vi "_read_mixer_params.vi"(10 "Control":T1={"GPIB_ATT"="28", "6501Dev#"=1, "GPIB_SP"="18", "GPIB_PM"="13", "GPIB_DSA"="11", "GPIB_DMM (TPD)"="23", "GPIB_MPI"="2", "mortor設定"=[{"Axis"=0, "ID"=0, "HIspeed"=200.0, "LOspeed"=100.0, "ACCEL(ms)"=100.0, "Sratio"=50.0, "フリーラン\n"=FALSE, "文字列"="DSB HOT/COLD"}, {"Axis"=1, "ID"=0, "HIspeed"=4.0, "LOspeed"=4.0, "ACCEL(ms)"=100.0, "Sratio"=50.0, "フリーラン\n"=TRUE, "文字列"="SubMM Att"}, {"Axis"=0, "ID"=0, "HIspeed"=200.0, "LOspeed"=100.0, "ACCEL(ms)"=100.0, "Sratio"=50.0, "フリーラン\n"=TRUE, "文字列"="MPI Port1"}, {"Axis"=1, "ID"=0, "HIspeed"=200.0, "LOspeed"=100.0, "ACCEL(ms)"=100.0, "Sratio"=50.0, "フリーラン\n"=TRUE, "文字列"="MPI Port2"}, {"Axis"=1, "ID"=0, "HIspeed"=200.0, "LOspeed"=100.0, "ACCEL(ms)"=100.0, "Sratio"=50.0, "フリーラン\n"=TRUE, "文字列"="gainComp"}], "DATAパス"=path "C:/Documents and Settings/?澤佳?/デスクトップ/data/プロトカ?トリッジ/110113_protoC4-9/110127_mixtest", "DBパス "=path "Z:/band10/Labview_ALMA/MIX95/test", "comment"="mix10test", "ColdCarts"="003601", "Th"=300.0, "Tc"=77.0, "Set_SIS_volt"=2.0999999046325684, "Offset"=0.0, "control"=0, "FreqLO"=874.0, "Set_Mag_Cur"=800.0, "MPI offset(mm)"=22.962, "HOT/COLD"=0} {"HOT/COLD" items=["DSB", "SBR (Cart.)", "GainComp", "SBR (MIX)"]; "control" items=["CLOSE LOOP", "OPEN LOOP", "Not Control"]}, 11 "Bias_LO_equip":T3={"Node address"=19, "CAN Interface"="CAN0", "Cartridge band"=10, "Slave Node in"={"Address"=19, "Serial Number"=[16, 71, 55, 76, 1, 8, 0, -15]}, "ObjHandle out"=89391168, "POL"=1, "sb"=1, "GPIB_SM (SIS S,V)"="24", "GPIB_DMM (SIS I)"="22", "GPIB_SM (MAG I) "="25", "GPIB_SG(LO)"="19", "GPIB_PW (PAMP) "="6", "GPIB_TMP1(8ch)"="12", "GPIB_TMP2(2ch)  "="13", "WCA_avg"=10, "Rsen"=10.0, "BiasModule"=1, "LOModule "=5, "WCA_LO_FREQ_SET"={"YTO Low freq. [GHz]"=14.42, "YTO High freq. [GHz]"=17.7, "Kvco"=1, "Lock Pol."=0, "SET LO FREQ"=96.22222, "Multiplier"=6.0, "YTO (HEX)"=2014, "YTO ( FREQ)"=16.033167, "NULL PLL INTEGRATOR"=FALSE}, "Res for"=0} {"Res for" items=["none", "series res", "parallel res"]; "WCA_LO_FREQ_SET"."YTO ( FREQ)" min=25 max=150 step=0.0001 format="%.3f"; "WCA_LO_FREQ_SET"."Multiplier" min=3 max=6 step=3; "WCA_LO_FREQ_SET"."SET LO FREQ" min=25 max=150 step=0.0001 format="%.3f"; "WCA_LO_FREQ_SET"."Lock Pol." items=["Lower", "Upper"]; "WCA_LO_FREQ_SET"."Kvco" items=["7.5MHz/V", "15MHz/V"]; "WCA_LO_FREQ_SET"."YTO High freq. [GHz]" format="%.3f"; "WCA_LO_FREQ_SET"."YTO Low freq. [GHz]" format="%.3f"; "LOModule" items=["Manual Gunn+PAMP"=0, "PLL GUNN+PAMP"=5, "B10Lab LO"=1, "WCA LO"=2, ""=3, "YIG発信器"=4, "none"=99]; "BiasModule" items=["B10Lab Bias"=0, "WCA BiasModule"=1, "none"=99]; "Slave Node in"."Serial Number" format="%.0x"; "Slave Node in"."Address" format="%.0x"; "Cartridge band" max=10 step=1; "Node address" format="%.0x"}) -> (3 "文字列":string="4.20, 874.00, 2011-02-04  16:25:42,  2.16, 48.9, 8.7,,,1,5,1, 2.10, 0.00, 800.00,0.58")   [LabVIEW 2017]
uses:
  WCA_NAOJ_sub_vi/WCA_Global.vi
panel:
  in  "CLNA_SET":T2={"CLNA State"=1, "SET POL0 LNA1 STAGE1 DRAIN V"=0.0, "SET POL0 LNA1 STAGE1 DRAIN C"=0.0, "SET POL0 LNA1 STAGE2 DRAIN V"=0.0, "SET POL0 LNA1 STAGE2 DRAIN C"=0.0, "SET POL0 LNA1 STAGE3 DRAIN V"=0.0, "SET POL0 LNA1 STAGE3 DRAIN C"=0.0} {"SET POL0 LNA1 STAGE3 DRAIN C" min=0 max=20 step=0.01 format="%.2f"; "SET POL0 LNA1 STAGE3 DRAIN V" min=0 max=3 step=0.01 format="%.2f"; "SET POL0 LNA1 STAGE2 DRAIN C" min=0 max=20 step=0.01 format="%.2f"; "SET POL0 LNA1 STAGE2 DRAIN V" min=0 max=3 step=0.01 format="%.2f"; "SET POL0 LNA1 STAGE1 DRAIN C" min=0 max=20 step=0.01 format="%.2f"; "SET POL0 LNA1 STAGE1 DRAIN V" min=0 max=3 step=0.01 format="%.2f"; "CLNA State" items=["Disabled", "Enabled"]}
  out "Link済み":bool=TRUE
  # "Vd [V]"
  # "Id [mA]"
  # "Stage 1"
  # "Stage 2"
  # "Stage 3"
  # "LO freq. [GHz]"
  # "YTO LOW\n/High Freq."
  # "ZERO Intgrtr"
  # "Node Address"
  # "Serial Number"
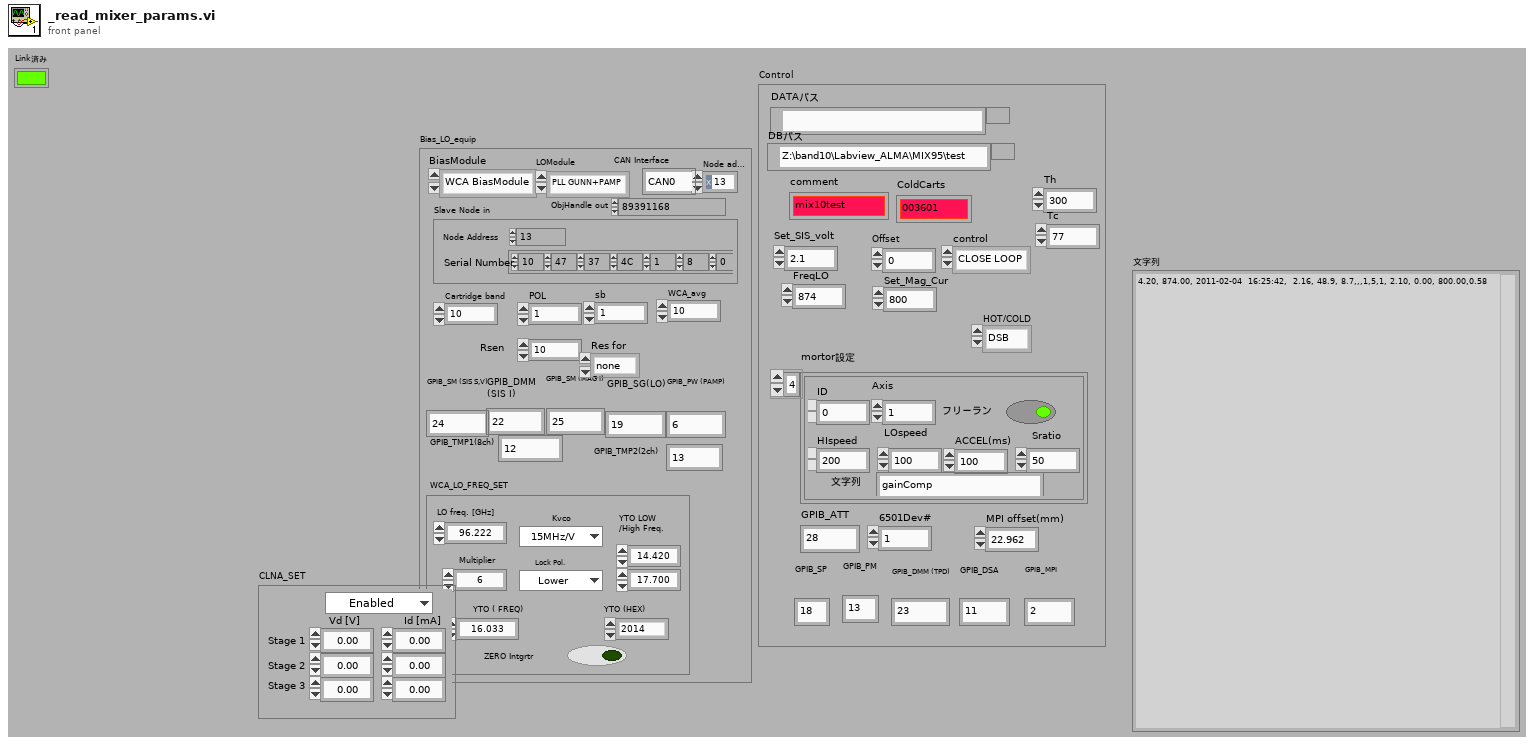
[diagram p1: front panel]
types:
  T1 = cluster{"GPIB_ATT":string, "6501Dev#":i16, "GPIB_SP":string, "GPIB_PM":string, "GPIB_DSA":string, "GPIB_DMM (TPD)":string, "GPIB_MPI":string, "mortor設定":cluster{"Axis":i16, "ID":i16, "HIspeed":dbl, "LOspeed":dbl, "ACCEL(ms)":dbl, "Sratio":dbl, "フリーラン\n":bool, "文字列":string}[], "DATAパス":path, "DBパス ":path, "comment":string, "ColdCarts":string, "Th":dbl, "Tc":dbl, "Set_SIS_volt":dbl, "Offset":dbl, "control":u16, "FreqLO":dbl, "Set_Mag_Cur":dbl, "MPI offset(mm)":dbl, "HOT/COLD":u16}
  T2 = cluster{"CLNA State":u8, "SET POL0 LNA1 STAGE1 DRAIN V":sgl, "SET POL0 LNA1 STAGE1 DRAIN C":sgl, "SET POL0 LNA1 STAGE2 DRAIN V":sgl, "SET POL0 LNA1 STAGE2 DRAIN C":sgl, "SET POL0 LNA1 STAGE3 DRAIN V":sgl, "SET POL0 LNA1 STAGE3 DRAIN C":sgl}
  T3 = cluster{"Node address":u16, "CAN Interface":string, "Cartridge band":u32, "Slave Node in":cluster{"Address":i16, "Serial Number":i8[]}, "ObjHandle out":u32, "POL":u32, "sb":u32, "GPIB_SM (SIS S,V)":string, "GPIB_DMM (SIS I)":string, "GPIB_SM (MAG I) ":string, "GPIB_SG(LO)":string, "GPIB_PW (PAMP) ":string, "GPIB_TMP1(8ch)":string, "GPIB_TMP2(2ch)  ":string, "WCA_avg":i32, "Rsen":dbl, "BiasModule":u16, "LOModule ":u16, "WCA_LO_FREQ_SET":cluster{"YTO Low freq. [GHz]":sgl, "YTO High freq. [GHz]":sgl, "Kvco":u16, "Lock Pol.":u16, "SET LO FREQ":sgl, "Multiplier":sgl, "YTO (HEX)":u16, "YTO ( FREQ)":sgl, "NULL PLL INTEGRATOR":bool}, "Res for":u16}
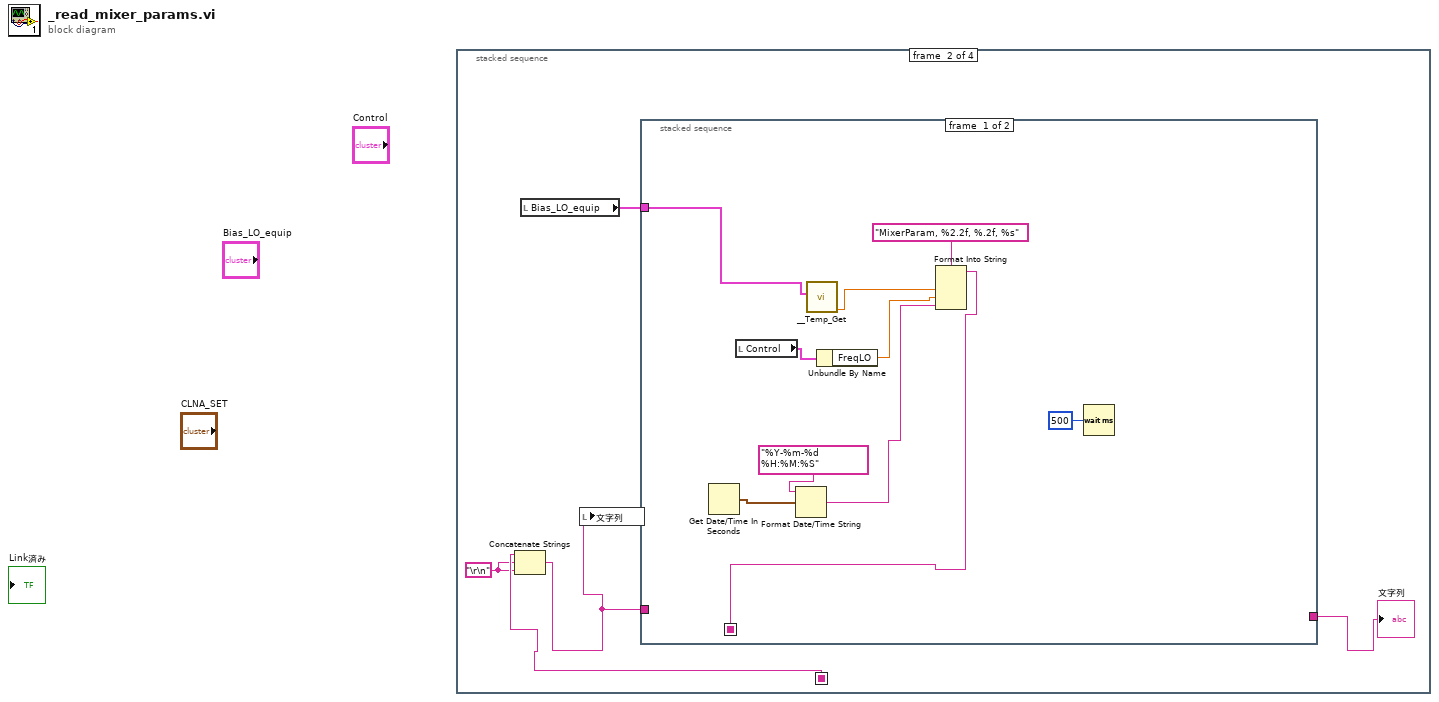
[diagram p0: block diagram]
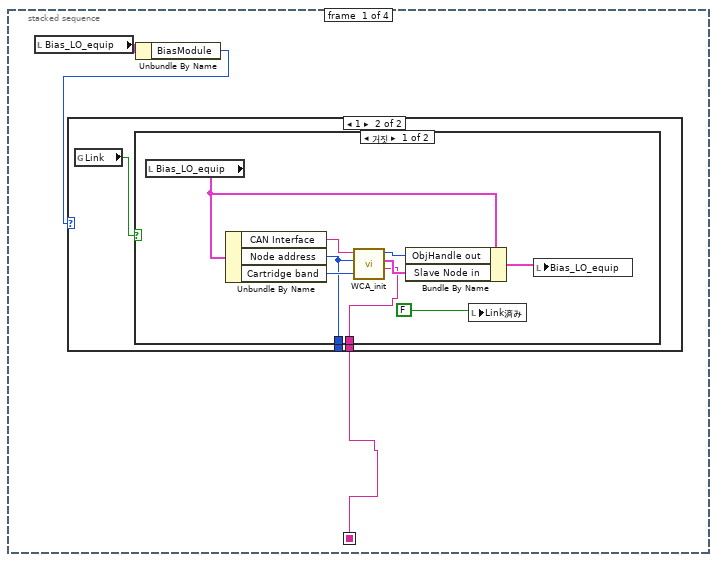
[diagram p2: hidden frame]
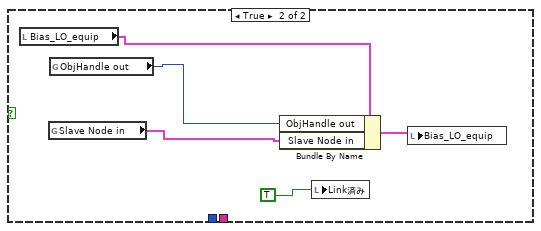
[diagram p4: hidden frame]
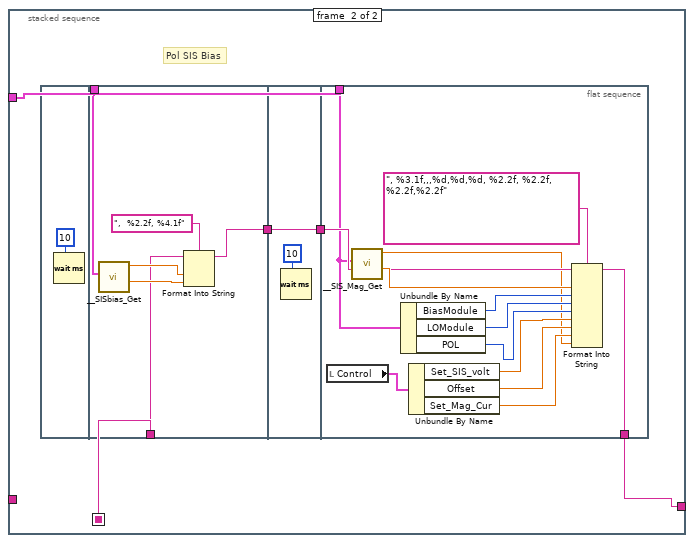
[diagram p5: hidden frame]
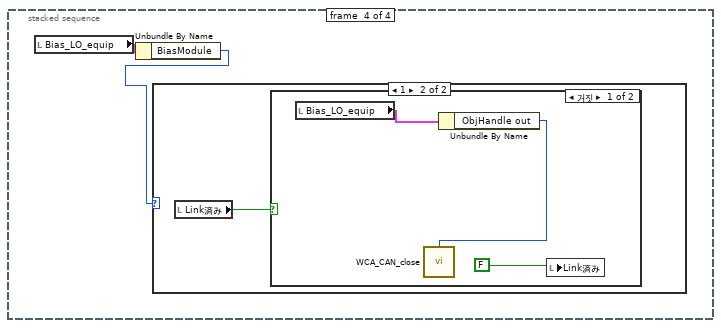
[diagram p7: hidden frame]
diagram:
  n1 = stacked-sequence {
    seq-local: [w1 _ _ _] -> [_ w24 _ _]
    frame #0 {
      n2 = local read "Bias_LO_equip"() -> (w3:T3)
      n3 = Unbundle By Name(w3) -> ("BiasModule"=w2:u16)
      n4 = case shown="1" w2 {
        tunnel: [_ w5] -> w1
        tunnel: [_ w4] -> _
        frame 0, Default {
        }
        frame 1 {
          n5 = global read "WCA_Global.vi" "Link"() -> (w6:bool)
          n6 = case shown="거짓" w6 {
            tunnel: [w7 _] -> w5
            tunnel: [w8 _] -> w4
            frame False {
              n7 = local read "Bias_LO_equip"() -> (w9:T3)
              n8 = Unbundle By Name(w9) -> ("CAN Interface"=w12:string, "Node address"=w8:u16, "Cartridge band"=w11:u32)
              n9 = call "WCA_init.vi"("Cartridge band"=w11, "Node address"=w8, "CAN Interface"=w12) -> ("Detected CAN Nodes."=w7:string, "Slave Node in"=w14:cluster{"Address":i16, "Serial Number":i8[]}, "ObjHandle out"=w15:u32)  [unwired: 4 in, 2 out]
              n10 = Bundle By Name(cluster=w9, "ObjHandle out"=w15, "Slave Node in"=w14) -> (w10:T3)
              n11 = local write "Link済み"(FALSE) -> ()
              n12 = local write "Bias_LO_equip"(w10) -> ()
            }
            frame True {
              n13 = local read "Bias_LO_equip"() -> (w19:T3)
              n14 = global read "WCA_Global.vi" "Slave Node in"() -> (w17:cluster{"Address":i16, "Serial Number":i8[]})
              n15 = global read "WCA_Global.vi" "ObjHandle out"() -> (w18:u32)
              n16 = Bundle By Name(cluster=w19, "ObjHandle out"=w18, "Slave Node in"=w17) -> (w20:T3)
              n17 = local write "Link済み"(TRUE) -> ()
              n18 = local write "Bias_LO_equip"(w20) -> ()
            }
          }
        }
      }
    }
    frame #1 {
      w23 = "\r\n"
      n19 = Concatenate Strings(w24, w23, w23) -> (w22:string)
      n20 = local read "Bias_LO_equip"() -> (w21:T3)
      n21 = local write "文字列"(w22) -> ()
      n22 = stacked-sequence {
        seq-local: [w26 _] -> [_ w40]
        tunnel: w22 -> [_ _]
        tunnel: [_ w36] -> w25
        tunnel: w21 -> [w34 w37]
        frame #0 {
          n23 = Get Date/Time In Seconds() -> (seconds since 1Jan1904=w31:timestamp)
          n24 = local read "Control"() -> (w29:T1)
          n25 = Format Date/Time String(time format string (%c)="%Y-%m-%d  %H:%M:%S", seconds (now)=w31) -> (date/time string=w27:string)  [unwired: 1 in]
          n26 = call "__Temp_Get.vi"("Bias_LO_equip"=w34) -> ("MixTemp"=w32:dbl)  [unwired: 8 in, 2 out]
          n27 = Unbundle By Name(w29) -> ("FreqLO"=w28:dbl)
          n28 = Format Into String(format string="MixerParam, %2.2f, %.2f, %s", w32, w28, w27) -> (resulting string=w26:string)  [unwired: 2 in, 1 out]
          n29 = Wait (ms)(milliseconds to wait=500) -> ()  [unwired: 1 out]
        }
        frame #1 {
          # "Pol SIS Bias"
          n30 = flat-sequence {
            tunnel: w37 -> [w46]
            tunnel: w40 -> [w43]
            tunnel: [w42] -> w38
            tunnel: [w48] -> w39
            tunnel: w38 -> [w48]
            tunnel: w39 -> [w60]
            tunnel: w37 -> [w59]
            tunnel: [w50] -> w36
            frame #0 {
              n31 = Wait (ms)(milliseconds to wait=10) -> ()  [unwired: 1 out]
            }
            frame #1 {
              n32 = call "__SISbias_Get.vi"("Bias_LO_equip"=w46) -> ("Get_I(uA)"=w44:dbl, "Get_V(mV)"=w45:dbl)  [unwired: 8 in, 1 out]
              n33 = Format Into String(format string=",  %2.2f, %4.1f", initial string=w43, w45, w44) -> (resulting string=w42:string)  [unwired: 1 in, 1 out]
            }
            frame #2 {
              n34 = Wait (ms)(milliseconds to wait=10) -> ()  [unwired: 1 out]
            }
            frame #3 {
              n35 = local read "Control"() -> (w55:T1)
              n36 = call "__SIS_Mag_Get.vi"("Bias_LO_equip"=w59) -> ("Get_Mag_I"=w61:dbl, "Get_Mag_V"=w51:dbl)  [unwired: 9 in]
              n37 = Unbundle By Name(w59) -> ("BiasModule"=w58:u16, "LOModule"=w57:u16, "POL"=w56:u32)
              n38 = Unbundle By Name(w55) -> ("Set_SIS_volt"=w54:dbl, "Offset"=w53:dbl, "Set_Mag_Cur"=w52:dbl)
              n39 = Format Into String(format string=", %3.1f,,,%d,%d,%d, %2.2f, %2.2f, %2.2f,%2.2f", initial string=w60, w61, w58, w57, w56, w54, w53, w52, w51) -> (resulting string=w50:string)  [unwired: 1 in, 1 out]
            }
          }
        }
      }
      "文字列" <- w25
    }
    frame #2 {
    }
    frame #3 {
      n40 = local read "Bias_LO_equip"() -> (w64:T3)
      n41 = Unbundle By Name(w64) -> ("BiasModule"=w63:u16)
      n42 = case shown="1" w63 {
        frame 0, Default {
        }
        frame 1 {
          n43 = local read "Link済み"() -> (w65:bool)
          n44 = case shown="거짓" w65 {
            frame False {
              n45 = local read "Bias_LO_equip"() -> (w67:T3)
              n46 = Unbundle By Name(w67) -> ("ObjHandle out"=w66:u32)
              n47 = call "WCA_CAN_close.vi"("ObjHandle in"=w66) -> ()  [unwired: 14 in, 1 out]
              n48 = local write "Link済み"(FALSE) -> ()
            }
            frame True {
            }
          }
        }
      }
    }
  }
